vi "Start.vi"(8 "error in (no error)":errorcluster, 11 "AODAcq in":refnum<class "AODAcq.lvclass">) -> (0 "error out":errorcluster, 3 "AODAcq out":refnum<class "AODAcq.lvclass">)   [LabVIEW 2011, in "AODAcq.lvclass"]
uses:
  AODAcq.lvclass
  AODAcq.lvclass/AODAcq.ctl
  <instrlib>/niHWS/nihws.llb/niHWS Set Wfm String Attribute ID.ctl
  <instrlib>/niHWS/nihws.llb/niHWS Set Wfm DBL Attribute.vi
  <vilib>/Utility/error.llb/Error Cluster From Error Code.vi
  <vilib>/rvi/errors/niLvFpgaAdjustHostInterfaceError.vi
  Program Files/National Instruments/LabVIEW 2011/Targets/NI/FPGA/StockFPGA_IntfPrivate/ScriptTemplates/StockFPGA_PlugInRead32.vi
  <vilib>/rvi/interface/nirviMethod/nirviMethod.xnode
  FPGA_Control/AODRef.ctl
  FPGA_Control/FPGA Bitfiles/AODControl_FPGATarget_5751Acquire_F1CF9257.lvbitx
  FPGA_Control/AOD Control (FPGA).vi
  <vilib>/rvi/interface/nirviReadWriteControl/nirviReadWriteControl.xnode
  <vilib>/FPGAPlugInAG/PXIe-7965R/niLvFpga_ReadFifo_PXIe-7965R.vi
  <vilib>/rvi/errors/niLvFpgaMergeErrorWithErrorCode.vi
  NiFpgaLv.dll
  <vilib>/FPGAPlugInAG/PXIe-7965R/niLvFpga_Read32_PXIe-7965R.vi
  <vilib>/rvi/interface/nirviReadWriteControl/niFpgaRWControlAccessTimeoutTemplate.vi
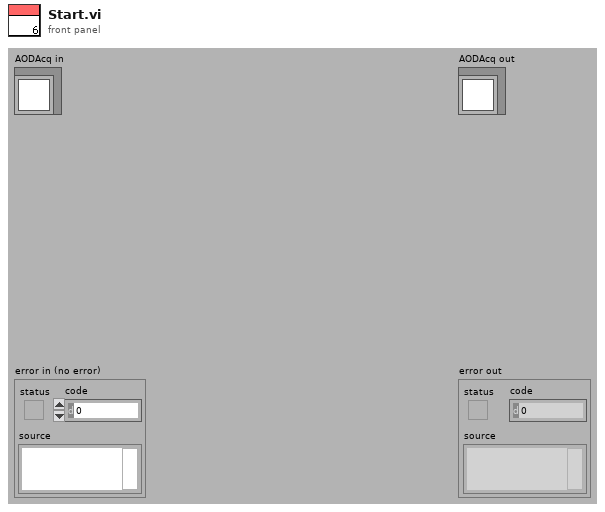
[diagram p1: front panel]
types:
  T1 = typedef "AODRef.ctl" = refnum<k20>
  T2 = typedef "niHWS Set Wfm String Attribute ID.ctl" = u32
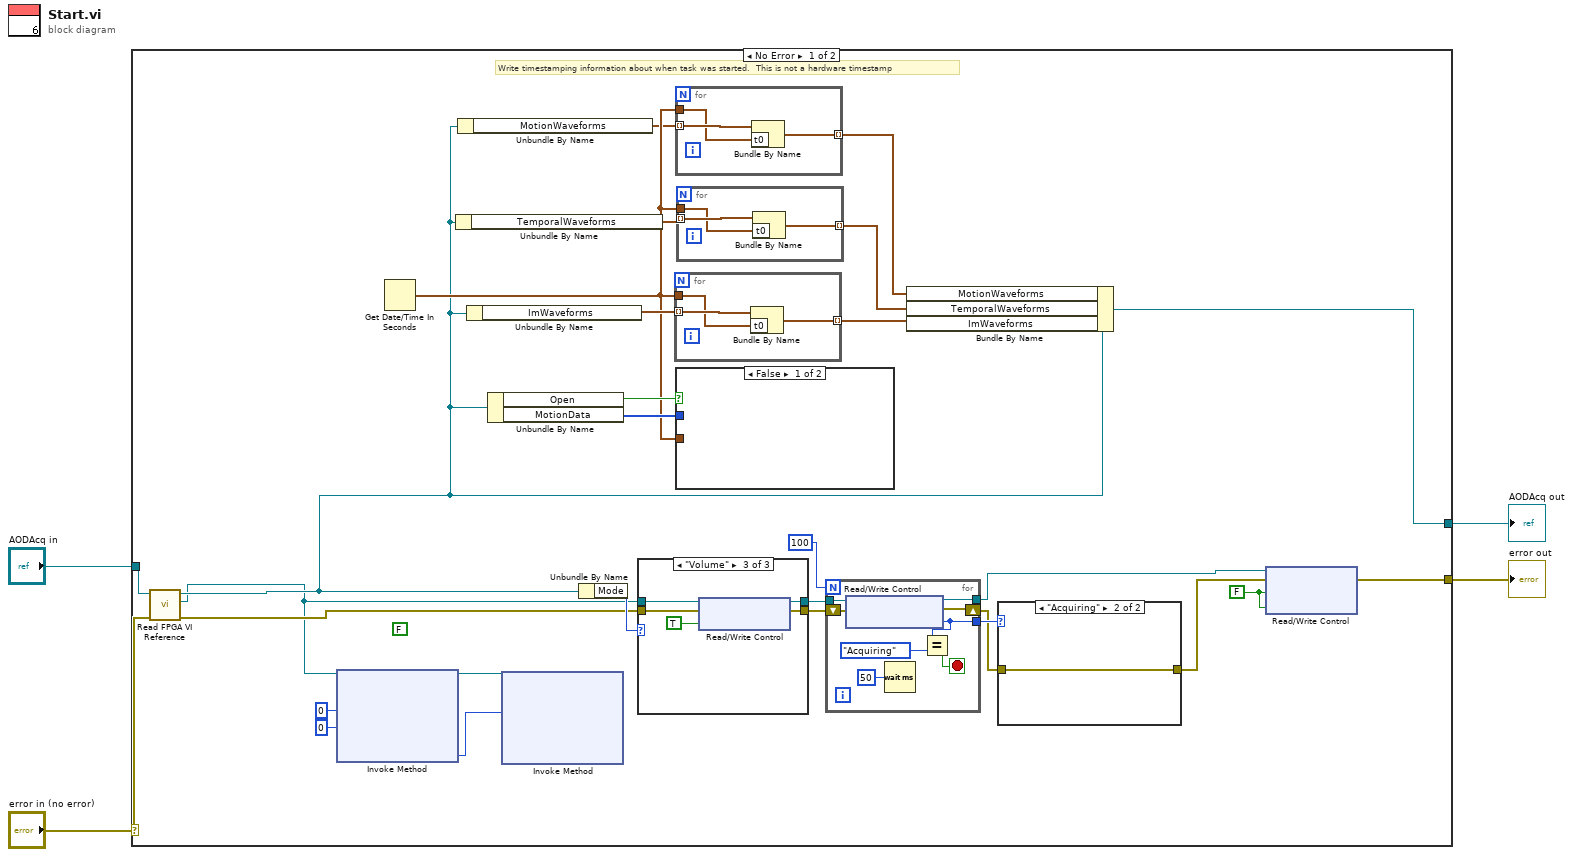
[diagram p0: block diagram]
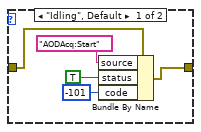
[diagram p2: hidden frame]
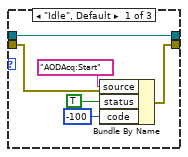
[diagram p3: hidden frame]
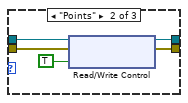
[diagram p4: hidden frame]
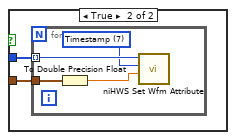
[diagram p5: hidden frame]
diagram:
  n1 = case shown="No Error" "error in (no error)" {
    selector: "error in (no error)" -> [w32 w80]
    tunnel: [w22 w80] -> w3
    tunnel: [w29 w79] -> w1
    tunnel: "AODAcq in" -> [w33 w79]
    frame No Error {
      w11 = FALSE ("ExtAcqTrig")
      (unwired) FALSE ("ExtAcqTrig")
      # "Write timestamping information about when task was started.  This is not a hardware timestamp"
      n2 = call-dynamic "Read FPGA VI Reference.vi"("error in (no error)"=w32, "AODAcq in"=w33) -> ("error out"=w10:errorcluster, "FPGA VI Reference"=w9:T1, "AODAcq out"=w12:refnum<class "AODAcq.lvclass">)  [unwired: 7 in]
      n3 = xnode "Invoke Method"("FPGA VI Reference In"=w9, "Number of Elements"=u32 0, "Timeout (ms)"=0) -> ("FPGA VI Reference Out"=w19:T1, "Elements Remaining"=w18:u32)  [unwired: 1 in, 2 out]
      n4 = Get Date/Time In Seconds() -> (seconds since 1Jan1904=w17:timestamp)
      n5 = Unbundle By Name(w12) -> ("TemporalWaveforms"=w16:waveform(i32)[])
      n6 = Unbundle By Name(w12) -> ("MotionWaveforms"=w15:waveform(i32)[])
      n7 = Unbundle By Name(w12) -> ("ImWaveforms"=w31:waveform(i32)[])
      n8 = Unbundle By Name(w12) -> ("Open"=w28:bool, "MotionData"=w27:u32[])
      n9 = xnode "Invoke Method"("FPGA VI Reference In"=w19, "Number of Elements"=w18) -> ()  [unwired: 2 in, 4 out]
      n10 = Unbundle By Name(w12) -> ("Mode"=w26:enum16{"Idle", "Points", "Volume"})
      n11 = case shown="\"Volume\"" w26 {
        tunnel: w9 -> [w59 w64 w68]
        tunnel: [w59 w63 w67] -> w23
        tunnel: [w55 w61 w66] -> w24
        tunnel: w10 -> [w54 w60 w65]
        frame "Idle", Default {
          n12 = Bundle By Name(cluster=w54, "source"="AODAcq:Start", "status"=TRUE, "code"=-100) -> (w55:errorcluster)
        }
        frame "Points" {
          n13 = xnode "Read/Write Control"("FPGA VI Reference In"=w64, "error in"=w60, "Control.Points"=TRUE) -> ("FPGA VI Reference Out"=w63:T1, "error out"=w61:errorcluster)
        }
        frame "Volume" {
          n14 = xnode "Read/Write Control"("FPGA VI Reference In"=w68, "error in"=w65, "Control.Volume"=TRUE ("Control.Points")) -> ("FPGA VI Reference Out"=w67:T1, "error out"=w66:errorcluster)
        }
      }
      n15 = for {
        tunnel: w31 -> [w78] mode=indexing
        tunnel: w17 -> [w77]
        tunnel: [w76] -> w30 mode=indexing
        n16 = Bundle By Name(cluster=w78, "t0"=w77) -> (w76:waveform(i32))
      }
      n17 = for {
        tunnel: w15 -> [w36] mode=indexing
        tunnel: w17 -> [w35]
        tunnel: [w34] -> w13 mode=indexing
        n18 = Bundle By Name(cluster=w36, "t0"=w35) -> (w34:waveform(i32))
      }
      n19 = case shown="False" w28 {
        tunnel: w27 -> [_ w71]
        tunnel: w17 -> [_ w70]
        frame False {
        }
        frame True {
          n20 = for {
            tunnel: w71 -> [w75] mode=indexing
            tunnel: w70 -> [w73]
            w74 = T2 7 items=["Note"=0, "X Axis Label"=1, "Y Axis Label"=2, "X Axis Units"=3, "Y Axis Units"=4, "Valid Signals"=6, "Timestamp"=7] ("attribute ID")
            n21 = To Double Precision Float(number=w73) -> (double precision float=w72:dbl)
            n22 = call-poly <instrlib>:"niHWS Set Wfm Attribute.vi"("attribute value"=w72, "attribute ID"=w74, "waveform reference in"=w75) -> ()  [unwired: 7 in, 2 out]
          }
        }
      }
      n23 = for {
        tunnel: w16 -> [w39] mode=indexing
        tunnel: w17 -> [w38]
        tunnel: [w37] -> w14 mode=indexing
        n24 = Bundle By Name(cluster=w39, "t0"=w38) -> (w37:waveform(i32))
      }
      n25 = for {
        N: 100 -> [_]
        tunnel: w23 -> [w53]
        tunnel: [w52] -> w6
        shift-right: [w46] -> w7
        shift-left: w24 -> [w50]
        tunnel: [w47] -> w8
        stop <- w48 stop-if-true
        n26 = xnode "Read/Write Control"("FPGA VI Reference In"=w53, "error in"=w50) -> ("FPGA VI Reference Out"=w52:T1, "error out"=w46:errorcluster, "Status.AcqState"=w47:enum16{"Idling", "Acquiring"})
        n27 = Wait (ms)(milliseconds to wait=u32 50) -> ()  [unwired: 1 out]
        n28 = Equal?(x=w47, y=enum16{"Idling", "Acquiring"}."Acquiring") -> (x = y?=w48:bool)
      }
      n29 = Bundle By Name(cluster=w12, "MotionWaveforms"=w13, "TemporalWaveforms"=w14, "ImWaveforms"=w30) -> (w29:refnum<class "AODAcq.lvclass">)
      n30 = case shown="\"Acquiring\"" w8 {
        tunnel: [w41 w45] -> w5
        tunnel: w7 -> [w40 w45]
        frame "Idling", Default {
          n31 = Bundle By Name(cluster=w40, "source"="AODAcq:Start", "status"=TRUE, "code"=-101) -> (w41:errorcluster)
        }
        frame "Acquiring" {
        }
      }
      n32 = xnode "Read/Write Control"("FPGA VI Reference In"=w6, "error in"=w5, "Control.Points"=w11, "Control.Volume"=w11) -> ("error out"=w22:errorcluster)  [unwired: 1 out]
    }
    frame Error {
    }
  }
  "error out" <- w3
  "AODAcq out" <- w1
